vi "Run State (Backup).vi"(8 "error in (no error)":errorcluster, 10 "Reset":bool, 11 "Stepper in":refnum<class "Stepper.lvclass">) -> (0 "error out":errorcluster, 3 "Stepper out":refnum<class "Stepper.lvclass">)   [LabVIEW 2015, in "Stepper.lvclass"]
uses:
  Stepper.lvclass
  Stepper.lvclass/Stepper.ctl
  <vilib>/ptbypt/NI_PtbyPt.lvlib
panel:
  in  "y 2":dbl=2.5e-08 format="%#_13g"
  in  "x":dbl=-1.0 format="%#_13g"
  in  "y":i32=4
  in  "delta":dbl=0.009000000000000001 format="%#_13g"
  in  "sample length":i32=12
  in  "PID":cluster{"P":dbl, "I":dbl, "D":dbl}={"P"=20.0, "I"=0.0, "D"=0.0}
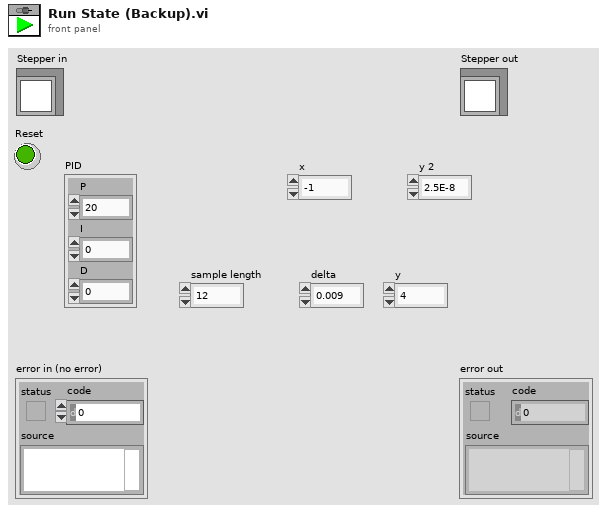
[diagram p1: front panel]
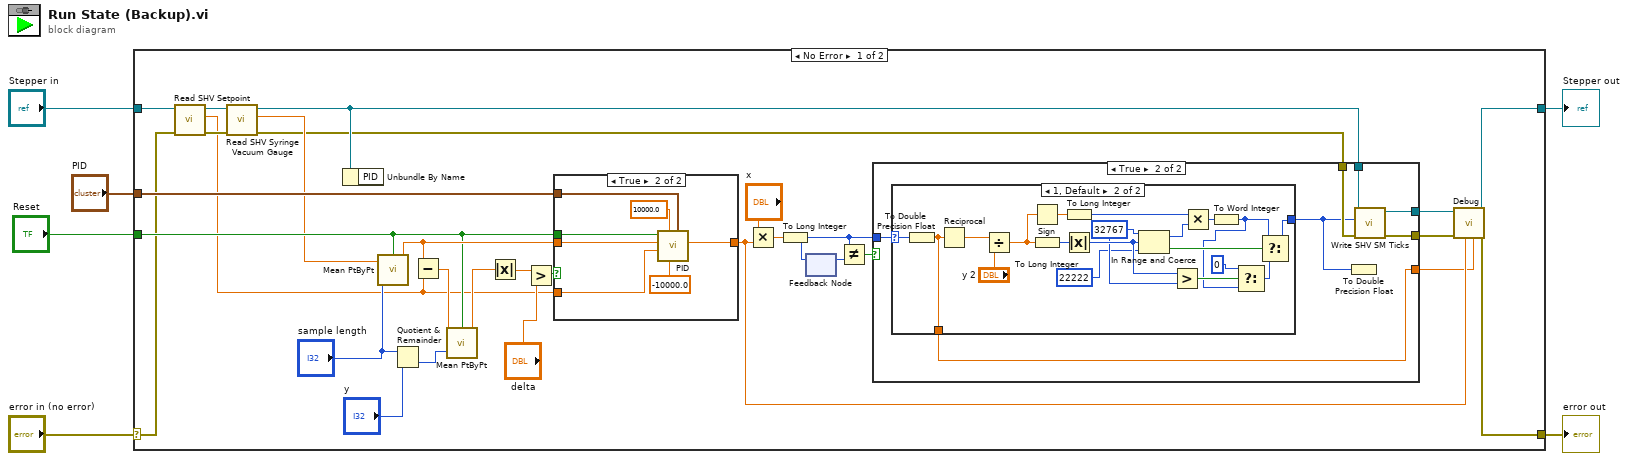
[diagram p0: block diagram]
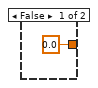
[diagram p2: hidden frame]
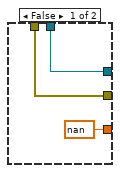
[diagram p3: hidden frame]
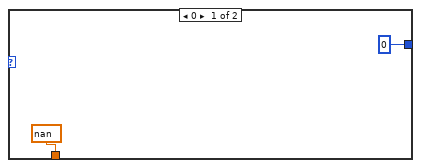
[diagram p4: hidden frame]
diagram:
  n1 = case shown="No Error" "error in (no error)" {
    selector: "error in (no error)" -> [w18 w77]
    tunnel: [w11 w77] -> w5
    tunnel: [w9 w76] -> w3
    tunnel: "Stepper in" -> [w20 w76]
    tunnel: "Reset" -> [w28 _]
    tunnel: "PID" -> [w32 _]
    frame No Error {
      n2 = call "Read SHV Setpoint.vi"("error in (no error)"=w18, "Stepper in"=w20) -> ("error out"=w17:errorcluster, "data out"=w16:dbl, "Stepper out"=w19:refnum<class "Stepper.lvclass">)  [unwired: 7 in]
      n3 = call "Read SHV Syringe Vacuum Gauge.vi"("error in (no error)"=w17, "Stepper in"=w19) -> ("error out"=w13:errorcluster, "Data"=w21:dbl, "Stepper out"=w14:refnum<class "Stepper.lvclass">)  [unwired: 7 in]
      n4 = Unbundle By Name(w14) -> ()  [unwired: 1 out]
      n5 = call <vilib>:"Mean PtByPt.vi"("x"=w21, "sample length"="sample length", "initialize"=w28) -> ("mean"=w31:dbl)  [unwired: 1 in, 1 out]
      n6 = Quotient & Remainder(x="sample length", y="y") -> (floor(x/y)=w24:i32)  [unwired: 1 out]
      n7 = Subtract(x=w31, y=w16) -> (x-y=w27:dbl)
      n8 = call <vilib>:"Mean PtByPt.vi"("x"=w27, "sample length"=w24, "initialize"=w28) -> ("mean"=w26:dbl)  [unwired: 1 in, 1 out]
      n9 = Absolute Value(x=w26) -> (abs(x)=w30:dbl)
      n10 = Greater?(x=w30, y="delta") -> (0:w29:bool)
      n11 = case shown="True" w29 {
        tunnel: [0.0 ("Output") w42] -> w8
        tunnel: w16 -> [_ w41]
        tunnel: w28 -> [_ w40]
        tunnel: w32 -> [_ w39]
        tunnel: w31 -> [_ w38]
        frame False {
        }
        frame True {
          n12 = call "PID.vi"("PID"=w39, "Lower Limit"=-10000.0, "Upper Limit (0,01)"=10000.0, "Setpoint (0,002)"=w41, "Process"=w38, "Reset"=w40) -> ("Output"=w42:dbl)  [unwired: 4 in, 1 out]
        }
      }
      n13 = Multiply(x="x", y=w8) -> (x*y=w15:dbl)
      n14 = To Long Integer(number=w15) -> (32bit integer=w34:i32)
      n15 = feedback #1() -> (w36:i32)  [unwired: 1 in]
      n16 = feedback-in #1(w34) -> ()
      n17 = Not Equal?(x=w34, y=w36) -> (x != y?=w35:bool)
      n18 = case shown="True" w35 {
        tunnel: w34 -> [_ w54]
        tunnel: w14 -> [w46 w53]
        tunnel: [w46 w52] -> w10
        tunnel: w13 -> [w47 w51]
        tunnel: [w47 w50] -> w12
        tunnel: [nan w48] -> w7
        frame False {
        }
        frame True {
          n19 = case shown="1, Default" w54 {
            selector: w54 -> [_ w74]
            tunnel: [i16 0 w62] -> w49
            tunnel: [nan w60] -> w48
            frame 0 {
            }
            frame 1, Default {
              w58 = 32767 ("upper limit")
              n20 = To Double Precision Float(number=w74) -> (double precision float=w60:dbl)
              n21 = Reciprocal(x=w60) -> (1/x=w69:dbl)
              n22 = Divide(x=w69, y="y 2") -> (x/y=w75:dbl)
              n23 = Sign(1:w75) -> (0:w72:dbl)
              n24 = To Long Integer(number=w75) -> (32bit integer=w73:i32)
              n25 = To Long Integer(number=w72) -> (32bit integer=w71:i32)
              n26 = Absolute Value(x=w73) -> (abs(x)=w59:i32)
              n27 = In Range and Coerce(upper limit=w58, x=w59, lower limit=22222) -> (coerced(x)=w65:i32, In Range?=w67:bool)
              n28 = Greater?(x=w59, y=w58) -> (0:w66:bool)
              n29 = Multiply(x=w71, y=w65) -> (x*y=w70:i32)
              n30 = To Word Integer(number=w70) -> (16bit integer=w61:i16)
              n31 = Select(t=i16 0, s=w66, f=w61) -> (s? t:f=w63:i16)
              n32 = Select(t=w61, s=w67, f=w63) -> (s? t:f=w62:i16)
            }
          }
          n33 = To Double Precision Float(number=w49) -> ()  [unwired: 1 out]
          n34 = call "Write SHV SM Ticks.vi"("error in (no error)"=w51, "Ticks (0)"=w49, "Stepper in"=w53) -> ("error out"=w50:errorcluster, "Stepper out"=w52:refnum<class "Stepper.lvclass">)  [unwired: 7 in]
        }
      }
      n35 = call "Debug.vi"("Numeric 1"=w7, "Numeric 0"=w8, "error in (no error)"=w12, "Stepper in"=w10) -> ("error out"=w11:errorcluster, "Stepper out"=w9:refnum<class "Stepper.lvclass">)  [unwired: 6 in]
    }
    frame Error {
    }
  }
  "error out" <- w5
  "Stepper out" <- w3
